vi "Image Trigger Global Count.vi"() -> ()   [LabVIEW 2019, in "Camera Controller.lvlib" / "Camera Controller.lvclass"]
uses:
  Camera Controller.lvclass
panel:
  in  "Image Trigger Count":u64
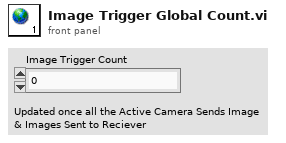
[diagram p1: front panel]
diagram:
